vi "TestGenericBinding.vi"() -> ()   [LabVIEW 2017]
uses:
  <vilib>/addons/InsightCM/MessageBus/Base/controls/MessageHeader.ctl
  <vilib>/addons/InsightCM/MessageBus/Base/controls/Message.ctl
  <vilib>/addons/InsightCM/MessageBus/Base/controls/KeyValuePair.ctl
panel:
  in  "MessageType":string
  out "Header 2":T1
  in  "Header":T1
  in  "stop":bool
  out "Received":string
  in  "Send":bool
  in  "MessageBody":string
  in  "BindingKey":string
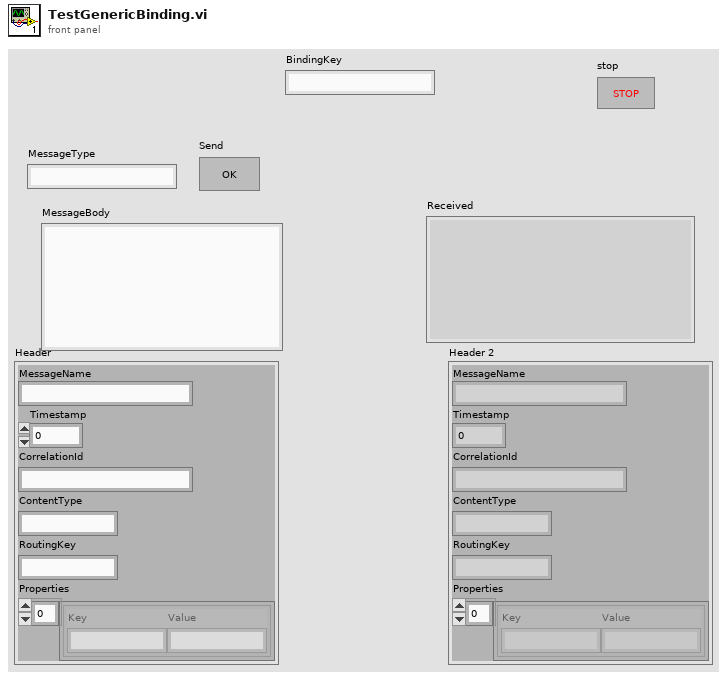
[diagram p1: front panel]
types:
  T1 = typedef "MessageHeader.ctl" = cluster{"MessageName":string, "Timestamp":i64, "CorrelationId":string, "ContentType":string, "RoutingKey":string, "Properties":T2[]}
  T2 = typedef "KeyValuePair.ctl" = cluster{"Key":string, "Value":string}
  T3 = typedef "MessageConsumer_Reference.ctl" = refnum<data-value>
  T4 = typedef "TcpMessageReference.ctl" = refnum<data-value>
  T5 = typedef "Message.ctl" = cluster{"Header":T1, "Body":u8[]}
  T6 = typedef "MessageHeader.ctl" = cluster{"MessageType":string, "Timestamp":i64, "CorrelationId":string, "ContentType":string, "Properties":cluster{"Key":string, "Value":string}[]}
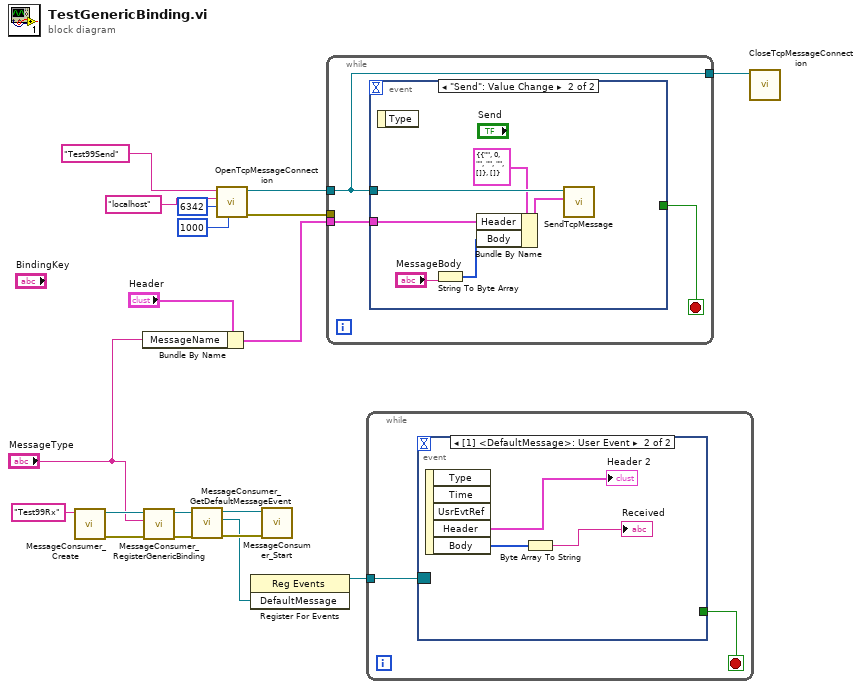
[diagram p0: block diagram]
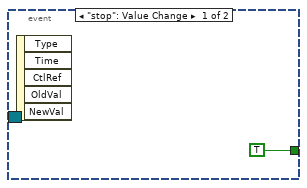
[diagram p2: hidden frame]
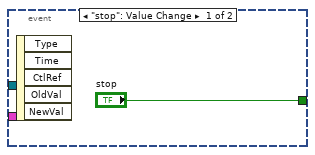
[diagram p3: hidden frame]
diagram:
  n1 = call <vilib>:"MessageConsumer_Create.vi"("ServiceName"="Test99Rx") -> ("error out"=w18:errorcluster, "Consumer"=w19:T3)  [unwired: 9 in]
  n2 = Bundle By Name(cluster="Header", "MessageName"="MessageType") -> (w1:T1)
  n3 = call <vilib>:"MessageConsumer_RegisterGenericBinding.vi"("error in (no error)"=w18, "BindingParameters"="MessageType", "Consumer"=w19) -> ("error out"=w15:errorcluster, "Consumer out"=w16:T3)  [unwired: 7 in]
  n4 = call <vilib>:"MessageConsumer_GetDefaultMessageEvent.vi"("error in (no error)"=w15, "Consumer"=w16) -> ("error out"=w14:errorcluster, "DefaultMessage"=w12:refnum<user-event>, "Consumer out"=w13:T3)  [unwired: 7 in]
  n5 = call <vilib>:"OpenTcpMessageConnection.vi"("timeout (ms)"=1000, "Port"=u16 6342, "Hostname"="localhost", "ClientName"="Test99Send" ("ServiceName")) -> ("error out"=w7:errorcluster, "connection ID out"=w6:T4)  [unwired: 6 in]
  n6 = register-events(w12) -> (reference out=w11:refnum<event-registration>)  [unwired: 2 in, 1 out]
  n7 = call <vilib>:"MessageConsumer_Start.vi"("error in (no error)"=w14, "Consumer"=w13) -> ()  [unwired: 8 in, 2 out]
  n8 = while {
    tunnel: w7 -> [_]
    tunnel: w6 -> [w21]
    tunnel: [w21] -> w5
    tunnel: w1 -> [w20]
    stop <- w22 stop-if-true
    n9 = event shown="[1] \"Send\": Value Change" {
      selector: _ -> [_ _]
      dyn-events: _ -> [_ _]
      timeout: _ -> [_ _]
      tunnel: ["stop" _] -> w22
      tunnel: w21 -> [_ w29]
      tunnel: w20 -> [_ w24]
      event "stop": Value Change {
        n10 = event-data() -> ()  [unwired: 1 in, 5 out]
      }
      event "Send": Value Change {
        n11 = event-data() -> ()  [unwired: 1 in, 1 out]
        n12 = String To Byte Array(string="MessageBody") -> (unsigned byte array=w25:u8[])
        n13 = Bundle By Name(cluster=T5 {"Header"={"MessageName"="", "Timestamp"=0, "CorrelationId"="", "ContentType"="", "RoutingKey"="", "Properties"=[]}, "Body"=[]} ("Message"), "Header"=w24, "Body"=w25) -> (w27:T5)
        n14 = call <vilib>:"SendTcpMessage.vi"("message"=w27, "connection ID in"=w29) -> ()  [unwired: 7 in, 3 out]
      }
    }
  }
  n15 = while {
    tunnel: w11 -> [w31]
    stop <- w30 stop-if-true
    n16 = event shown="[1] <DefaultMessage>: User Event" {
      selector: w31 -> [_ _]
      dyn-events: _ -> [_ _]
      timeout: _ -> [_ _]
      tunnel: [TRUE _] -> w30
      event "stop": Value Change {
        n17 = event-data() -> ()  [unwired: 1 in, 5 out]
      }
      event User Event {
        n18 = event-data() -> ("Header"=→"Header 2":T6, "Body"=w35:u8[])  [unwired: 1 in, 3 out]
        n19 = Byte Array To String(unsigned byte array=w35) -> (string=→"Received":string)
      }
    }
  }
  n20 = call <vilib>:"CloseTcpMessageConnection.vi"("connection ID in"=w5) -> ()  [unwired: 10 in, 1 out]
